vi "Main.vi"() -> ()   [LabVIEW 2015]
uses:
  Globals.vi
panel:
  in  "Services Token":string
  in  "Update Global":bool
  out "Global Slide Value":i32(slide) scale=0.0..100.0
  in  "Slide":i32(slide) scale=0.0..100.0
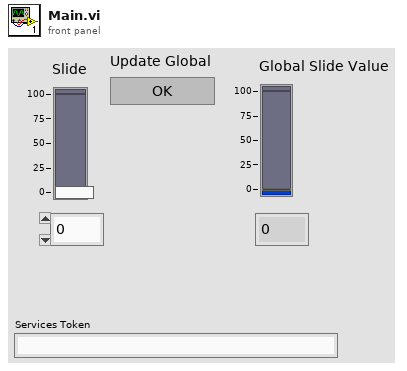
[diagram p1: front panel]
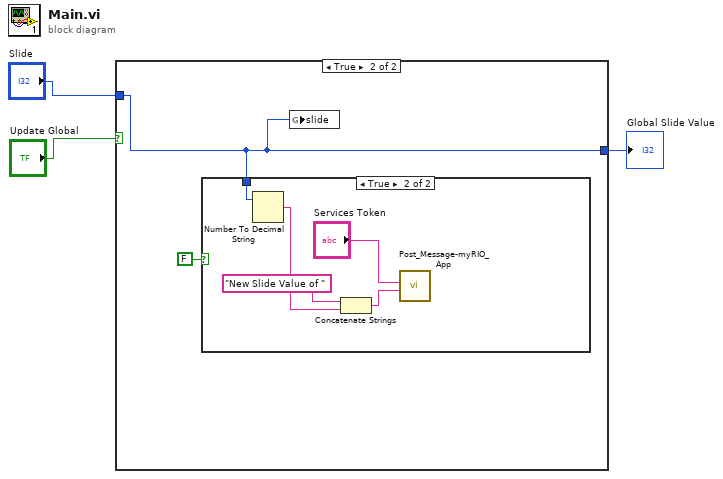
[diagram p0: block diagram]
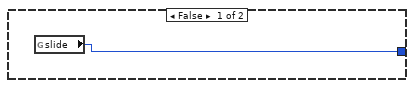
[diagram p2: hidden frame]
diagram:
  n1 = case shown="True" "Update Global" {
    tunnel: "Slide" -> [_ w6]
    tunnel: [w4 w6] -> w1
    frame False {
      n2 = global read "Globals.vi" "slide"() -> (w4:i32)
    }
    frame True {
      n3 = case shown="True" FALSE {
        tunnel: w6 -> [_ w11]
        frame False {
        }
        frame True {
          n4 = Number To Decimal String(number=w11) -> (decimal integer string=w10:string)  [unwired: 1 in]
          n5 = Concatenate Strings("New Slide Value of " ("string"), w10) -> (w8:string)
          n6 = call "Post_Message-myRIO_App.vi"("message"=w8, "Services Token"="Services Token") -> ()  [unwired: 8 in, 2 out]
        }
      }
      n7 = global write "Globals.vi" "slide"(w6) -> ()
    }
  }
  "Global Slide Value" <- w1
